vi "Formula_Node_Ejercicio.vi"() -> ()   [LabVIEW 2020]
panel:
  out "Gráfico de un circulo":cluster{dbl[], dbl[]}(graph)
  # "Diego Jáuregui Ontiveros\nCarlos Uriel Casas Casas\nAlejandro López González"
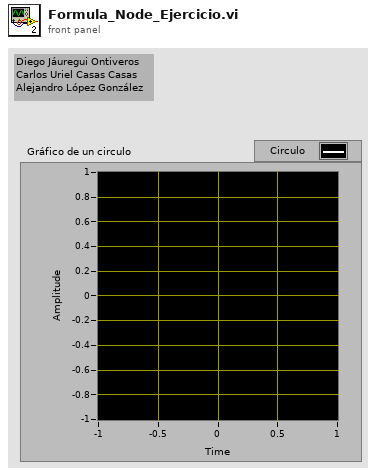
[diagram p1: front panel]
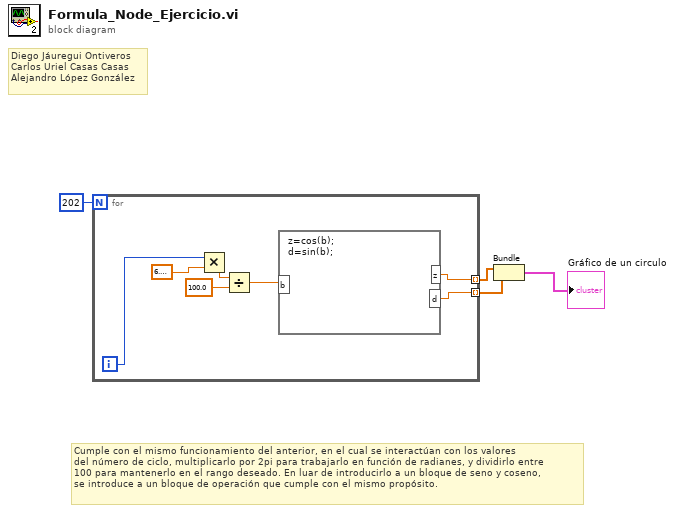
[diagram p0: block diagram]
diagram:
  # "Cumple con el mismo funcionamiento del anterior, en el cual se interactúan con los valores\ndel número de ciclo, multiplicarlo por 2pi para trabajarlo en función de radianes, y dividirlo entre\n100 para mantenerlo en el rango deseado. En luar de introducirlo a un bloque de seno y coseno,\nse introduce a un bloque de operación que cumple con el mismo propósito."
  # "Diego Jáuregui Ontiveros\nCarlos Uriel Casas Casas\nAlejandro López González"
  n1 = for {
    N: 202 -> [_]
    tunnel: [w6] -> w3 mode=indexing
    tunnel: [w5] -> w2 mode=indexing
    i -> [w11]
    n2 = Multiply(x=w11, y=6.283185307179586) -> (x*y=w9:dbl)
    n3 = Divide(x=w9, y=100.0) -> (x/y=w7:dbl)
    n4 = formula code="z=cos(b);\nd=sin(b);"("b"=w7) -> ("d"=w6:dbl, "z"=w5:dbl)
  }
  n5 = Bundle(w2, w3) -> (→"Gráfico de un circulo":cluster{dbl[], dbl[]})  [unwired: 1 in]
